vi "Report New State.vi"(8 "error in (no error)":errorcluster, 11 "Task in":refnum<class "Task.lvclass">) -> (0 "error out":errorcluster, 3 "Task out":refnum<class "Task.lvclass">)   [LabVIEW 2020, in "Volatus.lvlib" / "Task.lvclass"]
uses:
  Task.lvclass
  Task.lvclass/Task.ctl
  Event API/EventAPI.lvclass/EventAPI.ctl
  EventHandler Messages/Handle Event Msg/Handle Event Msg.lvclass/Handle Event Msg.ctl
  <vilib>/ActorFramework/Message Enqueuer/Message Enqueuer.lvclass/Message Enqueuer.ctl
  EventHandler Messages/Handle Event Msg/Send Handle Event.vi
  <vilib>/ActorFramework/Message Enqueuer/Enqueue.vi
  EventHandler Messages/Handle Event Msg/Handle Event Msg.lvclass
  C:/Program Files (x86)/National Instruments/LabVIEW 2020/vi.lib/ActorFramework/Message/Message.lvclass
  Task ID.vi
  <vilib>/ActorFramework/Message Priority Queue/Priority Enqueue.vi
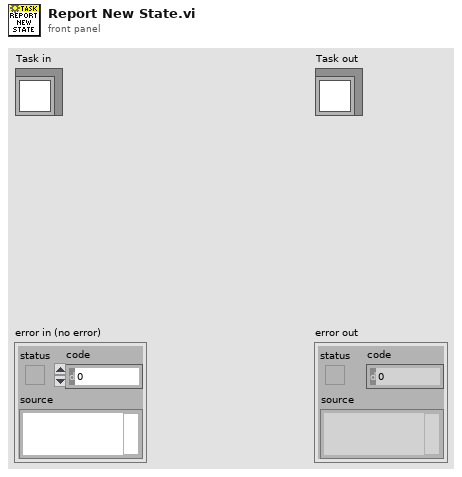
[diagram p1: front panel]
types:
  T1 = typedef "Volatus.lvlib/Task State.ctl" = enum16{"Unknown", "Idle", "Initializing", "Starting", "Running", "Stopping", "Stopped", "Error - Init", "Error - Start", "Error - Run", "Error - Stop"}
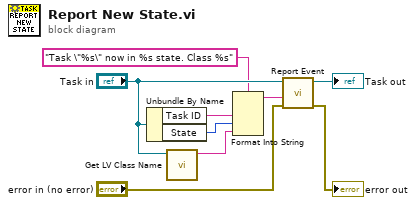
[diagram p0: block diagram]
diagram:
  n1 = Unbundle By Name("Task in") -> ("Task ID"=w7:string, "State"=w6:T1)
  n2 = call <vilib>:"Get LV Class Name.vi"("object"="Task in") -> ("class name"=w5:string)  [unwired: 9 in, 1 out]
  n3 = Format Into String(format string="Task \"%s\" now in %s state. Class %s", w7, w6, w5) -> (resulting string=w3:string)  [unwired: 2 in, 1 out]
  n4 = call "Report Event.vi"("error in (no error)"="error in (no error)", "Message"=w3, "Task in"="Task in") -> ("error out"=→"error out":errorcluster, "Task out"=→"Task out":refnum<class "Task.lvclass">)  [unwired: 7 in]
